vi "radiucenter2topleftwidthheight.vi"(6 "Radius":i32, 7 "ycenter":i32, 8 "xcenter":i32) -> (0 "Height":i32, 2 "Width":i32, 3 "Top":i32, 5 "Left":i32)   [LabVIEW 2019]
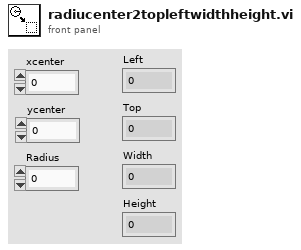
[diagram p1: front panel]
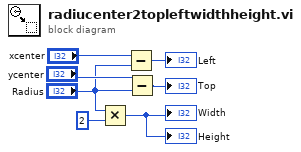
[diagram p0: block diagram]
diagram:
  n1 = Multiply(x="Radius", y=2) -> (x*y=→"Width" →"Height":i32)
  n2 = Subtract(x="xcenter", y="Radius") -> (x-y=→"Left":i32)
  n3 = Subtract(x="ycenter", y="Radius") -> (x-y=→"Top":i32)
